vi "RT_Read_Analog_Input_nw_check.vi"(8 "error in (no error)":errorcluster, 10 "Number Of Points":u32) -> (0 "error out":errorcluster, 3 "data read":bool, 5 "Data":fxp<+/-,17,5>[](array[numeric]))   [LabVIEW 2020]
uses:
  <vilib>/FPGAPlugInAG/cRIO-9040/niLvFpga_Open_cRIO-9040.vi
  <vilib>/Utility/error.llb/Error Cluster From Error Code.vi
  <vilib>/rvi/errors/niLvFpgaAdjustHostInterfaceError.vi
  <vilib>/rvi/interface/nirviOpenFPGA/nirviOpenFPGA.xnode
  FPGA Bitfiles/depapp_FPGATarget_FPGAmain_WC8wSYHNwdY.lvbitx
  FPGA_main.vi
  <vilib>/rvi/interface/nirviMethod/nirviMethod.xnode
  <vilib>/rvi/errors/niLvFpgaMergeErrorWithErrorCode.vi
  <vilib>/FPGAPlugInAG/cRIO-9040/niLvFpga_ReadFifo_cRIO-9040.vi
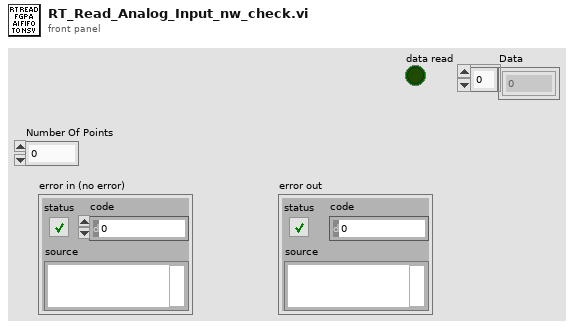
[diagram p1: front panel]
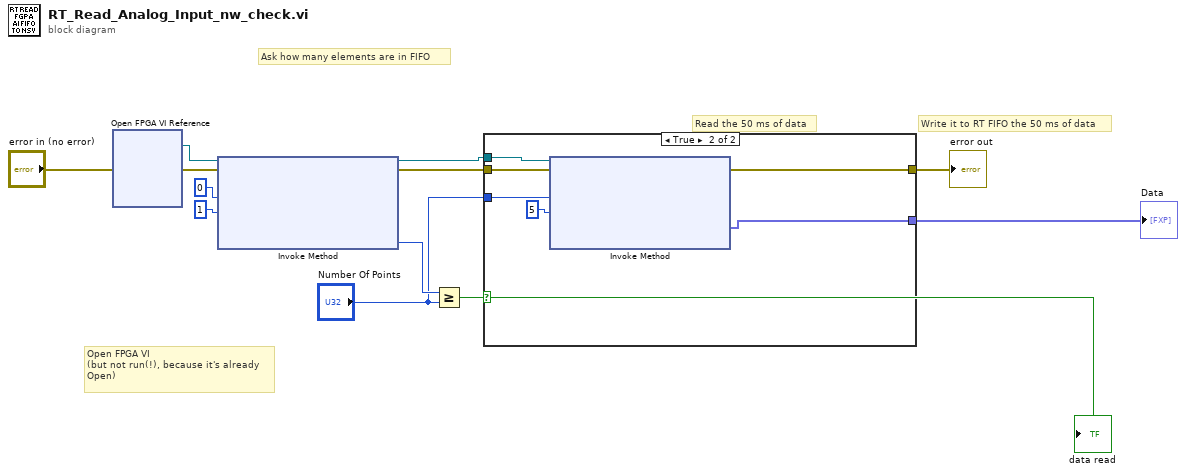
[diagram p0: block diagram]
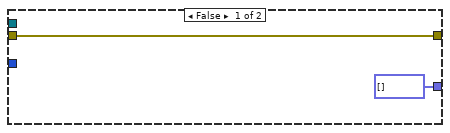
[diagram p2: hidden frame]
diagram:
  # "Write it to RT FIFO the 50 ms of data"
  # "Read the 50 ms of data"
  # "Ask how many elements are in FIFO"
  # "Open FPGA VI \n(but not run(!), because it's already \nOpen)"
  n1 = xnode "Open FPGA VI Reference"("error in"="error in (no error)") -> ("FPGA VI Reference Out"=w2:refnum<k20>, "error out"=w3:errorcluster)  [unwired: 1 in]
  n2 = xnode "Invoke Method"("FPGA VI Reference In"=w2, "error in"=w3, "Number of Elements"=u32 0, "Timeout (ms)"=1) -> ("FPGA VI Reference Out"=w10:refnum<k20>, "error out"=w11:errorcluster, "Elements Remaining"=w7:u32)  [unwired: 1 out]
  n3 = Greater Or Equal?(x=w7, y="Number Of Points") -> (x >= y?=w6:bool)
  "data read" <- w6
  n4 = case shown="True" w6 {
    tunnel: [w14 w20] -> w12
    tunnel: w11 -> [w14 w18]
    tunnel: w10 -> [_ w17]
    tunnel: "Number Of Points" -> [_ w16]
    tunnel: [fxp<+/-,17,5>[] [] ("Data") w15] -> w1
    frame False {
    }
    frame True {
      n5 = xnode "Invoke Method"("FPGA VI Reference In"=w17, "error in"=w18, "Number of Elements"=w16, "Timeout (ms)"=5) -> ("error out"=w20:errorcluster, "Data"=w15:fxp<+/-,17,5>[])  [unwired: 2 out]
    }
  }
  "error out" <- w12
  "Data" <- w1
